vi "SetLineStyle.vi"(0 "reference":refnum<class "StateTransitionEdge.lvclass">, 1 "lineStyle":refnum<class "LineStyle.lvclass">, 5 "error in (no error)":errorcluster) -> (14 "reference out":refnum<class "StateTransitionEdge.lvclass">, 19 "error out":errorcluster)   [LabVIEW 2020, in "StateTransitionEdge.lvclass"]
doc: "Sets the line style property.\n @param newValue the new value\n\n public void setLineStyle(LineStyle newValue)"
uses:
  <resource>/Framework/Providers/Open_GDS/UML/StateTransitionEdge_class/StateTransitionEdge.lvclass
  C:/Program Files (x86)/National Instruments/LabVIEW 2020/resource/Framework/Providers/Open_GDS/UML/SegmentedLineEdge_class/SegmentedLineEdge.lvclass
  <resource>/Framework/Providers/Open_GDS/UML/LineStyle_class/LineStyle.lvclass
  <resource>/Framework/Providers/Open_GDS/UML/SegmentedLineEdge_class/SegmentedLineEdge.lvclass
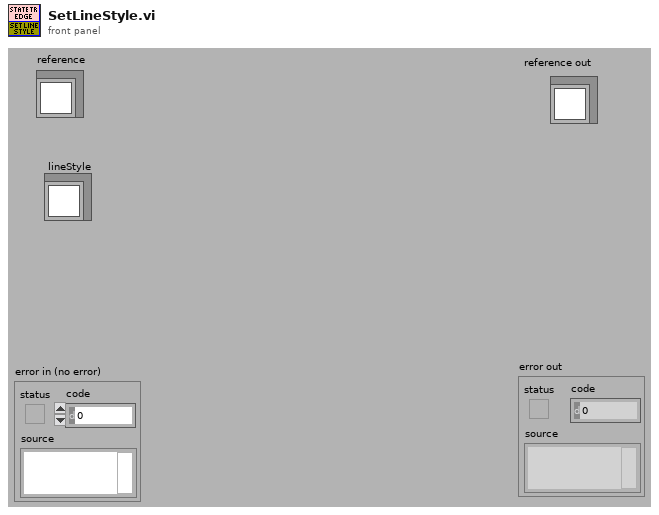
[diagram p1: front panel]
types:
  T1 = typedef "SegmentedLineEdge.lvclass/ObjectAttributes.ctl" = cluster{"lineStyle":refnum<class "LineStyle.lvclass">, "startArrowHead":refnum<class "ArrowHead.lvclass">, "endArrowHead":refnum<class "ArrowHead.lvclass">, "startLabel":string, "midLabel":string, "endLabel":string, "MidLabelOffset":T2, "SplitWire":bool}
  T2 = typedef "Point Point2D.ctl" = cluster{"x":dbl, "y":dbl}
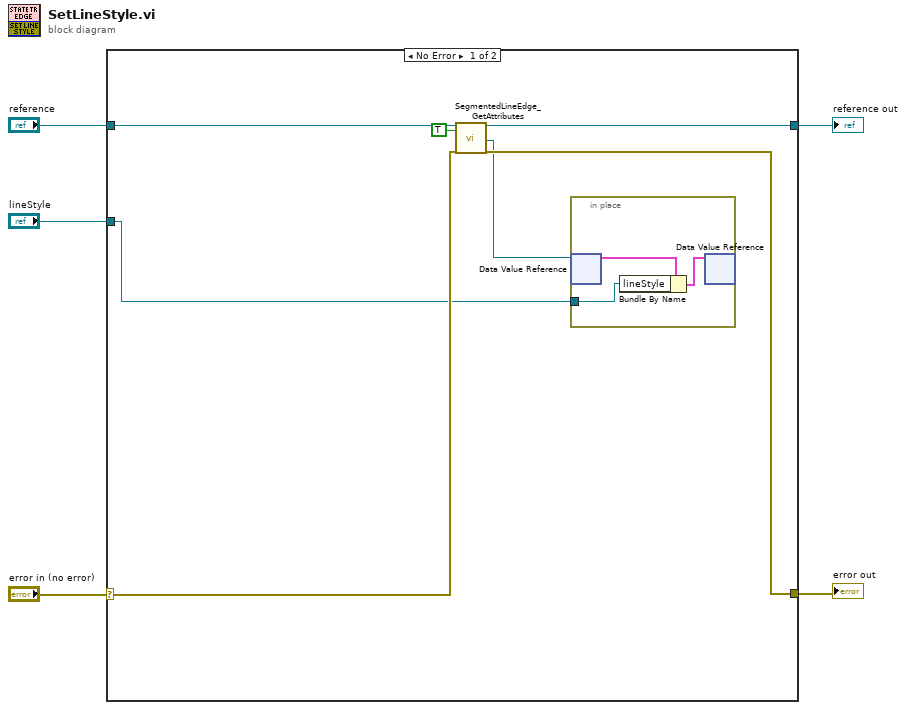
[diagram p0: block diagram]
diagram:
  n1 = case shown="No Error" "error in (no error)" {
    selector: "error in (no error)" -> [w9 w16]
    tunnel: "reference" -> [w12 w17]
    tunnel: [w11 w16] -> w4
    tunnel: [w10 w17] -> w3
    tunnel: "lineStyle" -> [w6 _]
    frame No Error {
      n2 = call <resource>:"SegmentedLineEdge_GetAttributes.vi"("reference in"=w12, "OnlyGetDvrReference(False)"=TRUE, "error in (no error)"=w9) -> ("reference out"=w10:refnum<class "StateTransitionEdge.lvclass">, "DataRef"=w7:refnum<data-value>, "error out"=w11:errorcluster)  [unwired: 13 in, 1 out]
      n3 = in-place {
        in-place-border: w6 -> [w14]
        n4 = in-place-dvr #1(w7) -> (w15:T1)  [unwired: 1 out]
        n5 = Bundle By Name(cluster=w15, "lineStyle"=w14) -> (w13:T1)
        n6 = in-place-dvr #1(w13) -> ()  [unwired: 2 out]
      }
    }
    frame Error {
    }
  }
  "reference out" <- w3
  "error out" <- w4
